vi "ConfigWindow.vi"(8 "error in (no error)":errorcluster) -> (0 "error out":errorcluster)   [LabVIEW 2015, in "ConfigHelper.lvlib"]
uses:
  ConfigHelper.lvlib
  Config.ctl
panel:
  in  "Days to Keep":i32=1 min=1 max=180 step=1
  in  "OK Button":bool
  in  "Cancel Button":bool
  in  "Export Folder Path":path
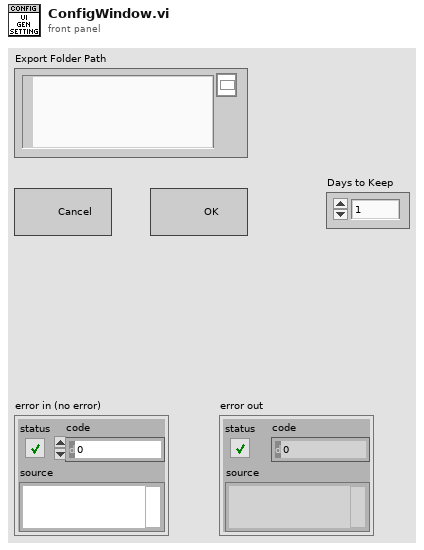
[diagram p1: front panel]
types:
  T1 = enum32{"Invalid", "Standard", "Closed", "Hidden", "Minimized", "Maximized"}
  T2 = typedef "ConfigHelper.lvlib/Config.ctl" = cluster{"Path":string, "Days to Keep":i32, "Number of Rows":i32}
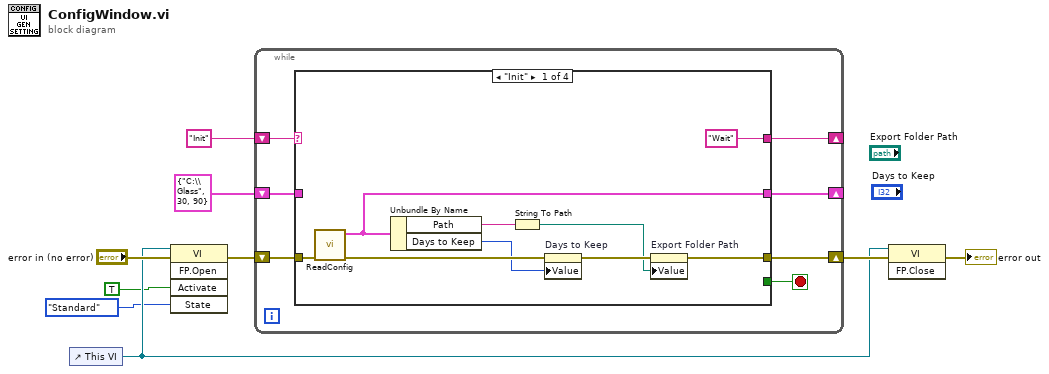
[diagram p0: block diagram]
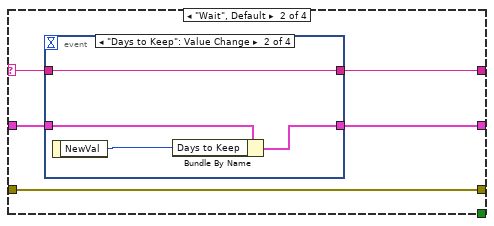
[diagram p2: hidden frame]
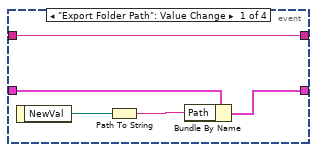
[diagram p3: hidden frame]
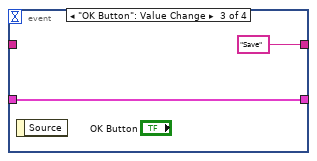
[diagram p4: hidden frame]
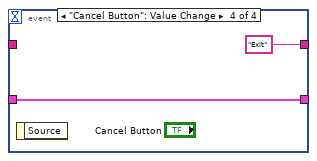
[diagram p5: hidden frame]
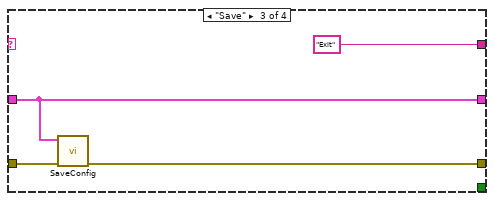
[diagram p6: hidden frame]
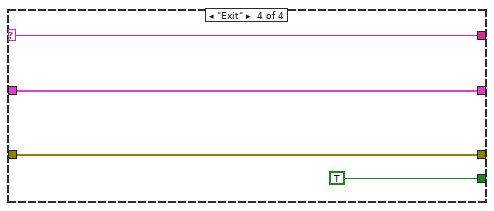
[diagram p7: hidden frame]
diagram:
  n1 = control-ref of="This VI"() -> (w3:refnum<vi>)
  n2 = invoke class="VI" method="FP.Open"(reference=w3, error in="error in (no error)", "Activate"=TRUE ("Activate?"), "State"=T1."Standard") -> (error out=w5:errorcluster)  [unwired: 1 in, 4 out]
  n3 = while {
    shift-right: [w12] -> _
    shift-left: "Init" -> [w16]
    shift-right: [w13] -> _
    shift-left: T2 {"Path"="C:\\Glass", "Days to Keep"=30, "Number of Rows"=90} ("Config") -> [w15]
    shift-right: [w11] -> w7
    shift-left: w5 -> [w14]
    stop <- w10 stop-if-true
    n4 = case shown="\"Init\"" w16 {
      selector: w16 -> [_ w30 _ w49]
      tunnel: w15 -> [_ w28 w46 w50]
      tunnel: w14 -> [w25 w26 w47 w51]
      tunnel: [w23 w27 w46 w50] -> w13
      tunnel: ["Wait" w29 "Exit" w49] -> w12
      tunnel: [w22 w26 w44 w51] -> w11
      tunnel: [_ _ _ TRUE] -> w10
      frame "Init" {
        n5 = call "ReadConfig.vi"("error in (no error)"=w25) -> ("error out"=w21:errorcluster, "Config"=w23:T2)  [unwired: 9 in]
        n6 = Unbundle By Name(w23) -> ("Path"=w18:string, "Days to Keep"=w19:i32)
        n7 = String To Path(string=w18) -> (path=w17:path)
        n8 = property on="Days to Keep" class="DigNum (strict)"(error in=w21, "Value"=w19) -> (error out=w20:errorcluster)  [unwired: 1 in, 1 out]
        n9 = property on="Export Folder Path" class="Path"(error in=w20, "Value"=w17) -> (error out=w22:errorcluster)  [unwired: 1 in, 1 out]
      }
      frame "Wait", Default {
        n10 = event shown="[1] \"Days to Keep\": Value Change" {
          selector: _ -> [_ _ _ _]
          dyn-events: _ -> [_ _ _ _]
          timeout: _ -> [_ _ _ _]
          tunnel: w30 -> [w35 w39 _ _]
          tunnel: [w35 w39 "Save" "Exit"] -> w29
          tunnel: w28 -> [w34 w38 w40 w42]
          tunnel: [w31 w37 w40 w42] -> w27
          event "Export Folder Path": Value Change {
            n11 = event-data() -> ("NewVal"=w33:path)  [unwired: 1 in]
            n12 = Path To String(path=w33) -> (string=w32:string)
            n13 = Bundle By Name(cluster=w34, "Path"=w32) -> (w31:T2)
          }
          event "Days to Keep": Value Change {
            n14 = event-data() -> ("NewVal"=w36:i32)  [unwired: 1 in]
            n15 = Bundle By Name(cluster=w38, "Days to Keep"=w36) -> (w37:T2)
          }
          event "OK Button": Value Change {
            n16 = event-data() -> ()  [unwired: 1 in, 1 out]
          }
          event "Cancel Button": Value Change {
            n17 = event-data() -> ()  [unwired: 1 in, 1 out]
          }
        }
      }
      frame "Save" {
        n18 = call "SaveConfig.vi"("error in (no error)"=w47, "Config"=w46) -> ("error out"=w44:errorcluster)  [unwired: 9 in]
      }
      frame "Exit" {
      }
    }
  }
  n19 = invoke class="VI" method="FP.Close"(reference=w3, error in=w7) -> (error out=→"error out":errorcluster)  [unwired: 1 in, 2 out]
